vi "Aero Cooling Global.vi"() -> ()   [LabVIEW 2022 SP3]
panel:
  in  "Minimum Value":dbl
  out "Ready?":bool=TRUE
  in  "Dem Pos %":dbl
  in  "Meas Pos %":dbl
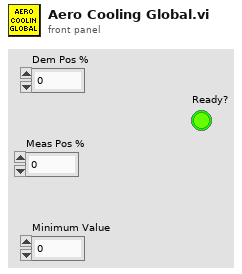
[diagram p1: front panel]
diagram:
